vi "Create.vi"(8 "error in (no error)":errorcluster, 10 "Folder Name":string, 11 "Hostname":string) -> (0 "error out":errorcluster, 3 "Folder Creation out":refnum<class "Folder Creation.lvclass">)   [LabVIEW 2014, in "Folder Creation.lvclass"]
uses:
  Folder Creation.lvclass
  Build Job/Build Job.lvclass/Build Job.ctl
  Build Job/Write Script Job Name.vi
  Build Job/Write Hostname.vi
  Build Job/Write Parameters.vi
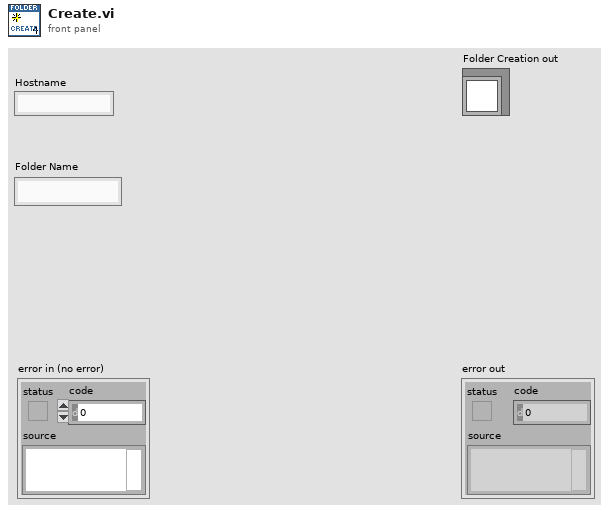
[diagram p1: front panel]
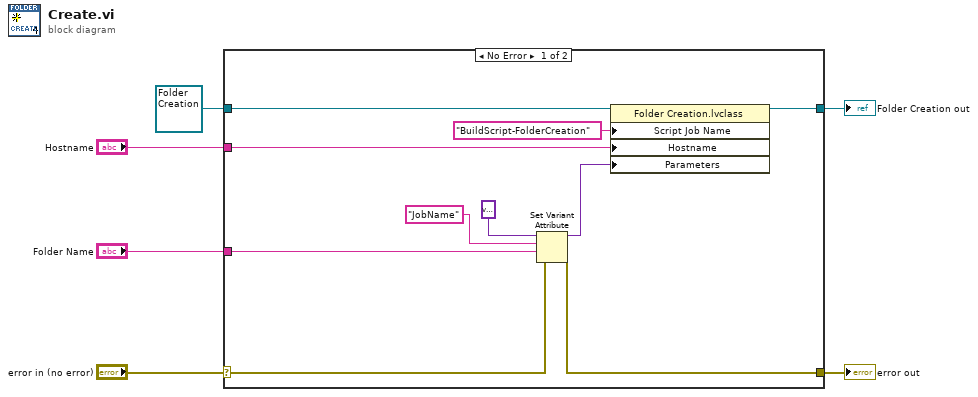
[diagram p0: block diagram]
diagram:
  n1 = case shown="No Error" "error in (no error)" {
    selector: "error in (no error)" -> [w9 w18]
    tunnel: [w8 w18] -> w5
    tunnel: [w15 w17] -> w3
    tunnel: refnum<class "Folder Creation.lvclass"> refnum ("Folder Creation in") -> [w16 w17]
    tunnel: "Hostname" -> [w13 _]
    tunnel: "Folder Name" -> [w7 _]
    frame No Error {
      n2 = Set Variant Attribute(Variant=variant ("variant"), name="JobName" ("Name"), value=w7, error in=w9) -> (Variant out=w10:variant, error out=w8:errorcluster)  [unwired: 1 out]
      n3 = property class="Folder Creation.lvclass"(reference=w16, "Script Job Name"="BuildScript-FolderCreation", "Hostname"=w13, "Parameters"=w10) -> (reference out=w15:refnum<class "Folder Creation.lvclass">)  [unwired: 1 in, 1 out]
    }
    frame Error {
    }
  }
  "error out" <- w5
  "Folder Creation out" <- w3
